vi "Fast Set Multiple Dependent Node Refs FuncGlobal.vi"(5 "Action":enum16{"Open or Add", "Close Ref"}(ring), 8 "error in (no error)":errorcluster, 9 "Dependent Node Refs":T1[](array[typedef]) format="%.0x", 10 "Base Property Name":string, 11 "Item Ref in":T1 format="%.0x") -> (0 "error out":errorcluster, 3 "Item Ref out":T1=18446744073709551615 format="%.0x")   [LabVIEW 2011]
uses:
  <vilib>/NI Veristand/Custom Device API/Custom Device Item Ref.ctl
  <vilib>/NI Veristand/Custom Device API/Set Item Property (Variant).vi
  <vilib>/NI Veristand/Custom Device API/Custom Device API.lvlib
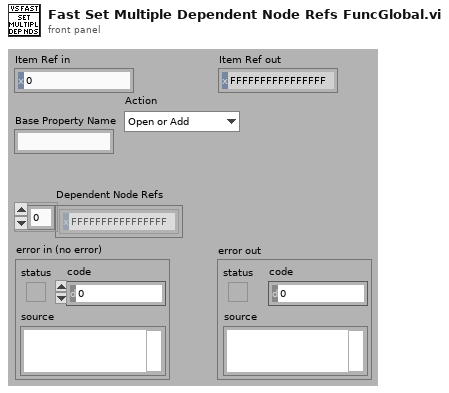
[diagram p1: front panel]
types:
  T1 = typedef "Custom Device API.lvlib/Custom Device Item Ref.ctl" = u64
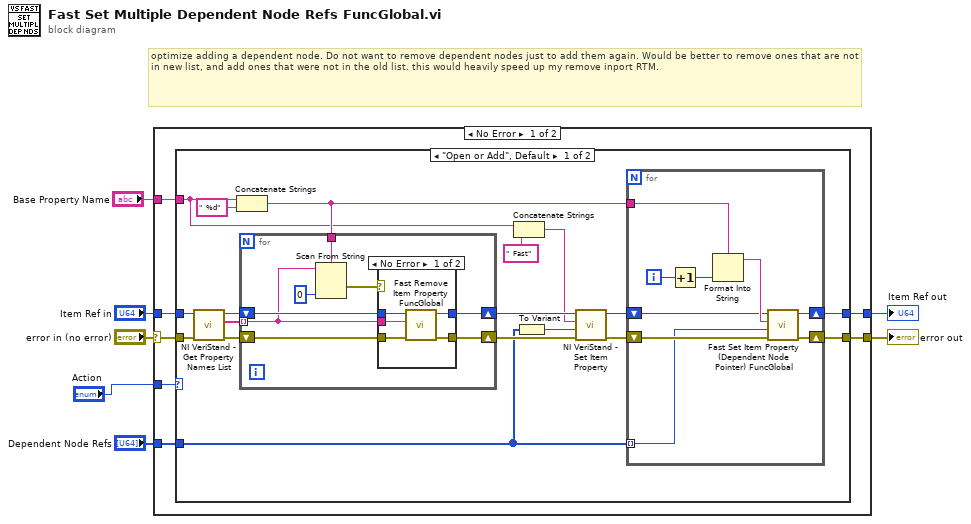
[diagram p0: block diagram]
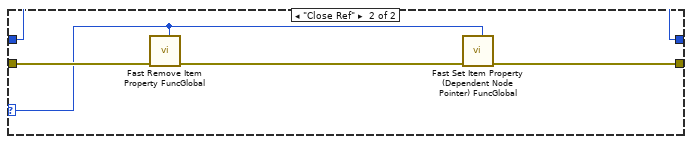
[diagram p3: hidden frame]
diagram:
  # "optimize adding a dependent node. Do not want to remove dependent nodes just to add them again. Would be better to remove ones that are not in new list, and add ones that were not in the old list. this would heavily speed up my remove inport RTM."
  n1 = case shown="No Error" "error in (no error)" {
    selector: "error in (no error)" -> [w9 w62]
    tunnel: "Item Ref in" -> [w14 w63]
    tunnel: "Dependent Node Refs" -> [w13 _]
    tunnel: [w12 w63] -> w5
    tunnel: [w11 w62] -> w4
    tunnel: "Base Property Name" -> [w10 _]
    tunnel: "Action" -> [w8 _]
    frame No Error {
      n2 = case shown="\"Open or Add\", Default" w8 {
        selector: w8 -> [_ w60]
        tunnel: w14 -> [w32 w57]
        tunnel: w13 -> [w16 _]
        tunnel: [w28 w57] -> w12
        tunnel: [w27 w58] -> w11
        tunnel: w10 -> [w15 _]
        tunnel: w9 -> [w25 w61]
        frame "Open or Add", Default {
          n3 = call <vilib>:"NI VeriStand - Get Property Names List.vi"("error in (no error)"=w25, "Item Ref in"=w32) -> ("error out"=w30:errorcluster, "Property Names"=w29:string[], "Item Ref out"=w31:T1)  [unwired: 7 in]
          n4 = Concatenate Strings(w15, "  %d" ("string")) -> (w23:string)
          n5 = for {
            shift-right: [w45] -> w22
            shift-left: w30 -> [w47]
            tunnel: w29 -> [w46] mode=indexing
            shift-right: [w44] -> w20
            shift-left: w31 -> [w49]
            tunnel: w23 -> [w43]
            n6 = Scan From String(format string=w43, input string=w46, default 1=0 ("default value 1")) -> (error out=w48:errorcluster)  [unwired: 3 in, 2 out]
            n7 = case shown="No Error" w48 {
              tunnel: w49 -> [w52 w55]
              tunnel: w47 -> [w54 w56]
              tunnel: w46 -> [w53 _]
              tunnel: [w50 w56] -> w45
              tunnel: [w51 w55] -> w44
              frame No Error {
                n8 = call "Fast Remove Item Property FuncGlobal.vi"("error in (no error)"=w54, "Property Name"=w53, "Item Ref in"=w52) -> ("error out"=w50:errorcluster, "Item Ref out"=w51:T1)  [unwired: 6 in, 1 out]
              }
              frame Error {
              }
            }
          }
          n9 = Concatenate Strings(w15, "  Fast" ("string")) -> (w18:string)
          n10 = To Variant(anything=w16) -> (Variant=w17:variant)
          n11 = call-poly <vilib>:"NI VeriStand - Set Item Property.vi"("error in (no error)"=w22, "Value"=w17, "Property Name"=w18, "Item Ref in"=w20) -> ("error out"=w21:errorcluster, "Item Ref out"=w19:T1)  [unwired: 5 in, 1 out]
          n12 = for {
            shift-right: [w33] -> w27
            shift-left: w21 -> [w38]
            tunnel: w23 -> [w40]
            shift-right: [w34] -> w28
            shift-left: w19 -> [w35]
            tunnel: w16 -> [w37] mode=indexing
            i -> [w41]
            n13 = Increment(x=w41) -> (x+1=w39:i32)
            n14 = Format Into String(format string=w40, w39) -> (resulting string=w36:string)  [unwired: 2 in, 1 out]
            n15 = call "Fast Set Item Property (Dependent Node Pointer) FuncGlobal.vi"("error in (no error)"=w38, "Dependent Node Ref"=w37, "Property Name"=w36, "Item Ref in"=w35) -> ("error out"=w33:errorcluster, "Item Ref out"=w34:T1)  [unwired: 5 in, 1 out]
          }
        }
        frame "Close Ref" {
          n16 = call "Fast Remove Item Property FuncGlobal.vi"("Action"=w60, "error in (no error)"=w61) -> ("error out"=w59:errorcluster)  [unwired: 7 in, 2 out]
          n17 = call "Fast Set Item Property (Dependent Node Pointer) FuncGlobal.vi"("Action"=w60, "error in (no error)"=w59) -> ("error out"=w58:errorcluster)  [unwired: 7 in, 2 out]
        }
      }
    }
    frame Error {
    }
  }
  "Item Ref out" <- w5
  "error out" <- w4
